vi "TopLevelController.vi"(8 "error in (no error)":errorcluster) -> (0 "error out":errorcluster)   [LabVIEW 2013, in "ToplevelControllerLibrary.lvlib"]
doc: "This Controller controls all interface (User,Display and Sensor )connected to it. New Interfaces can be added."
uses:
  ToplevelControllerLibrary.lvlib
  Modules/DisplayConsole/PrivateContols/DisplayConsole_QueueDriver.ctl
  Modules/UserConsole/PrivateControls/UserConsole_QueueDriver.ctl
  Modules/SensorConsole/PrivateControls/SensorConsole_QueueDriver.ctl
  Modules/Config Database/Private Controls/Queue Driver Control_Config DB.ctl
  Private Controls/Terminate.ctl
  Modules/SensorConsole/SensorConsoleLib.lvlib
  Modules/UserConsole/UserConsole.lvlib
  Modules/DisplayConsole/DisplayConsoleLib.lvlib
  Modules/Config Database/ConfigDBLib.lvlib
panel:
  # "This Controller controls all interface (User,Display and Sensor )connected to it. New Interfaces can be added."
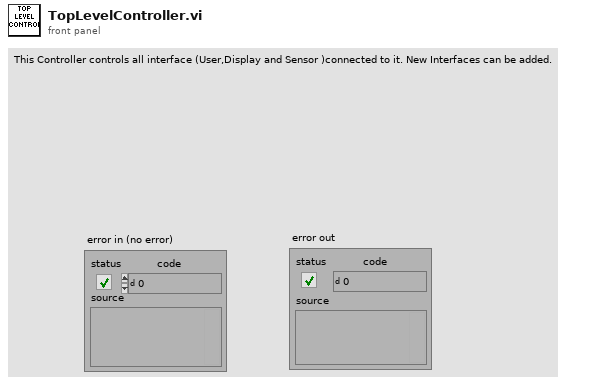
[diagram p1: front panel]
types:
  T1 = enum16{"Init", "Enqueue", "Dequeue", "ReleaseQueue", "Exit"}
  T2 = enum16{"Create Event", "Generate Event", "Destroy Event"}
  T3 = typedef "SensorConsoleLib.lvlib/SensorConsole_QueueDriver.ctl" = enum16{"Default case", "Init", "Enqueue", "Dequeue", "ReleaseQueue", "Exit"}
  T4 = typedef "UserConsole.lvlib/UserConsole_QueueDriver.ctl" = enum16{"Default Case", "Init", "Enqueue", "Dequeue", "ReleaseQueue", "Exit"}
  T5 = typedef "DisplayConsoleLib.lvlib/DisplayConsole_QueueDriver.ctl" = enum16{"Default Case", "Init", "Enqueue", "Dequeue", "ReleaseQueue", "Exit"}
  T6 = typedef "ConfigDBLib.lvlib/Queue Driver Control_Config DB.ctl" = enum16{"Init", "Enqueue", "Dequeue", "ReleaseQueue", "Exit"}
  T7 = typedef "ToplevelControllerLibrary.lvlib/Terminate.ctl" = enum16{"Update UserConsole", "Update DisplayConsole", "ReInit"}
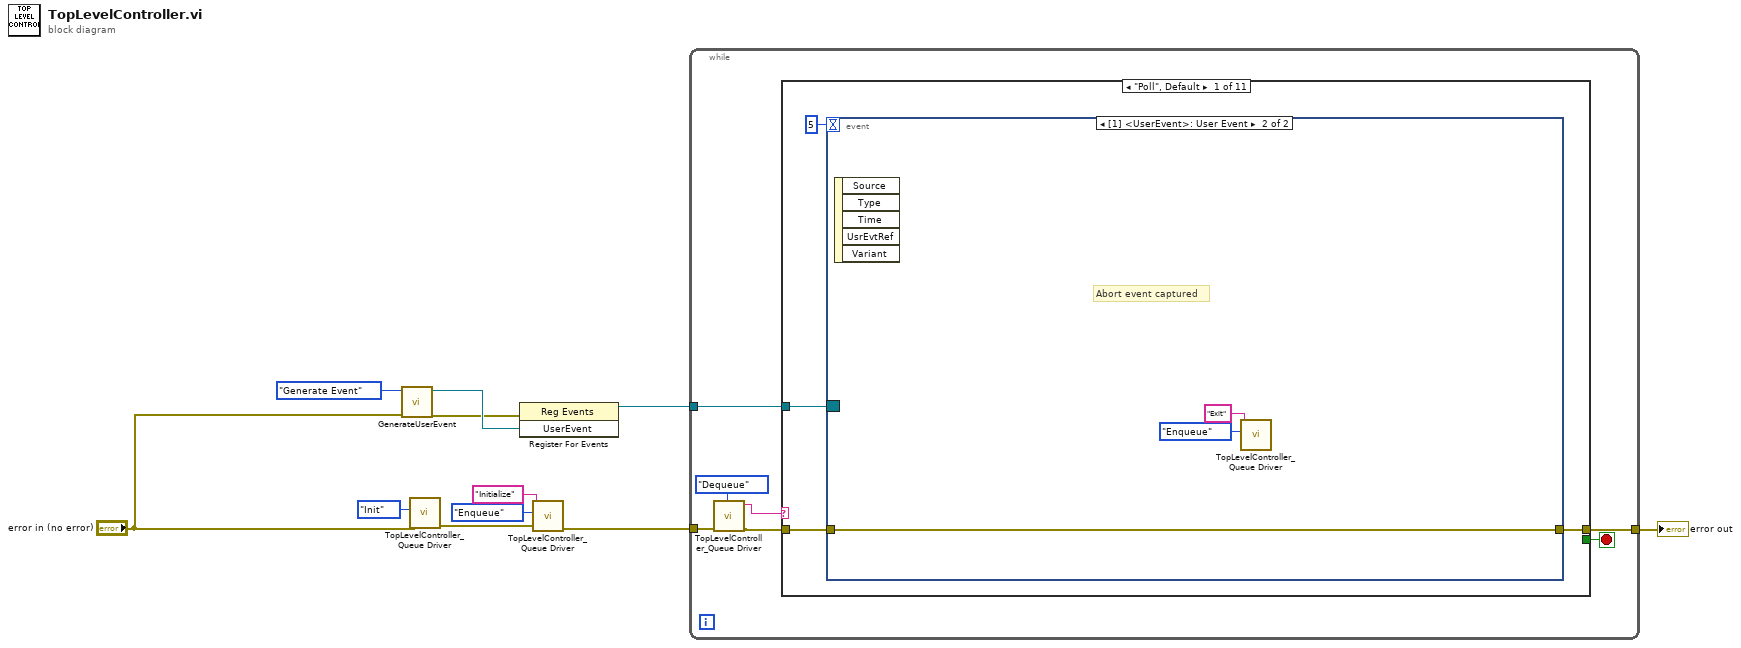
[diagram p0: block diagram]
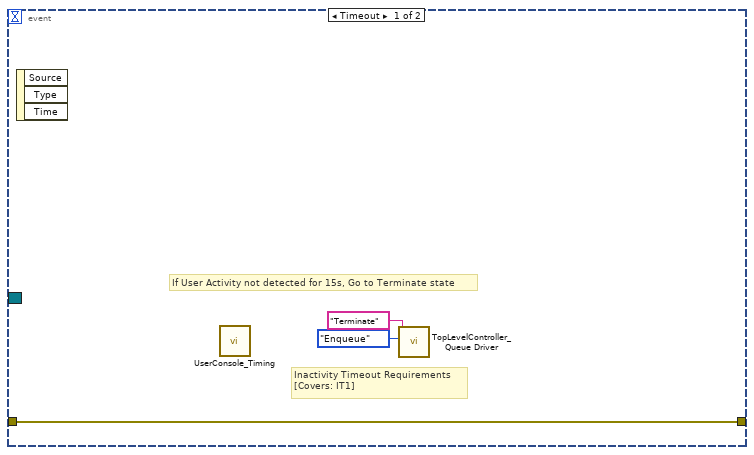
[diagram p2: hidden frame]
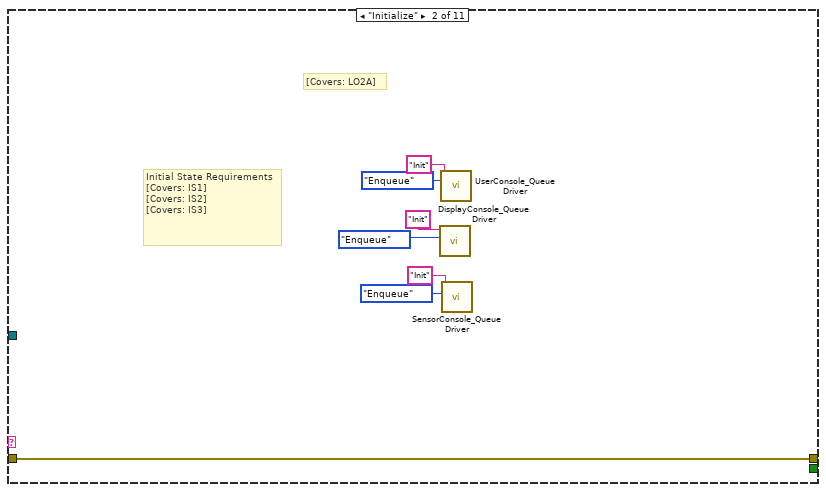
[diagram p3: hidden frame]
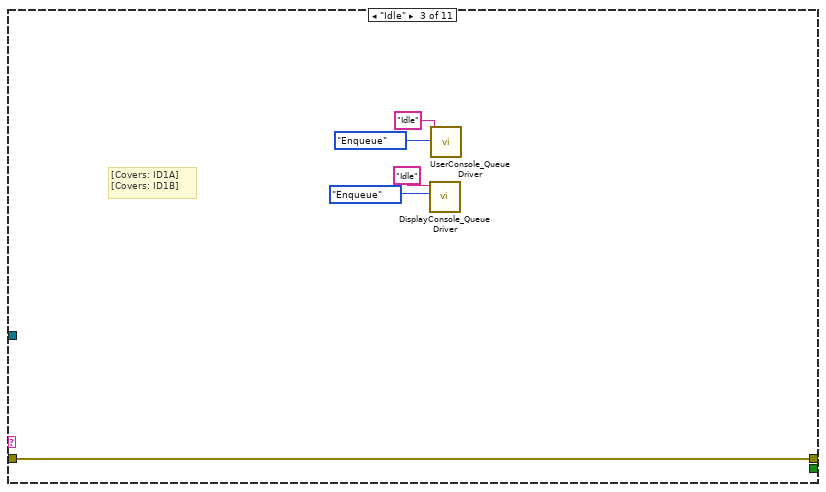
[diagram p4: hidden frame]
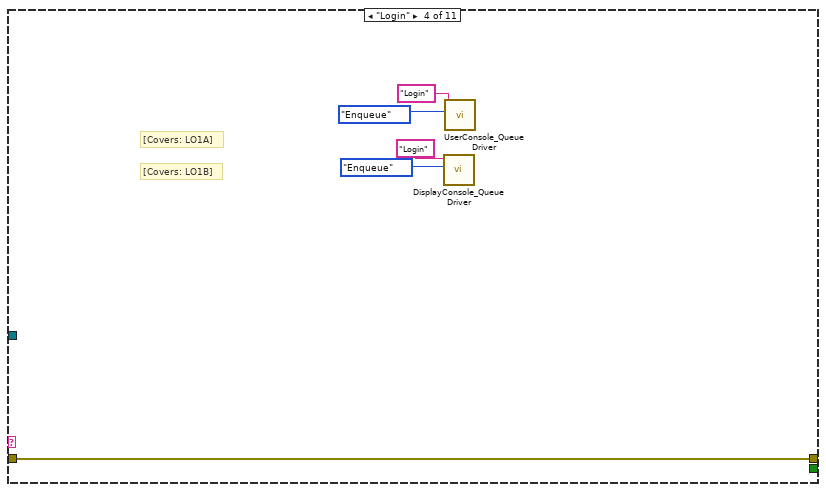
[diagram p5: hidden frame]
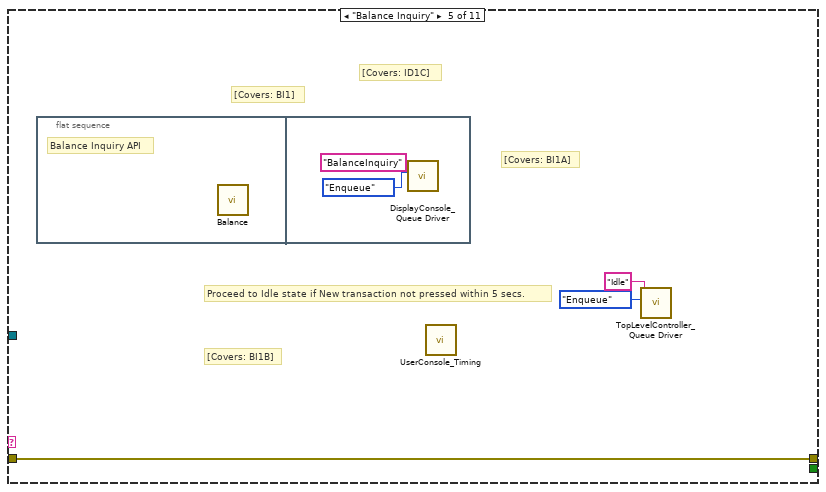
[diagram p6: hidden frame]
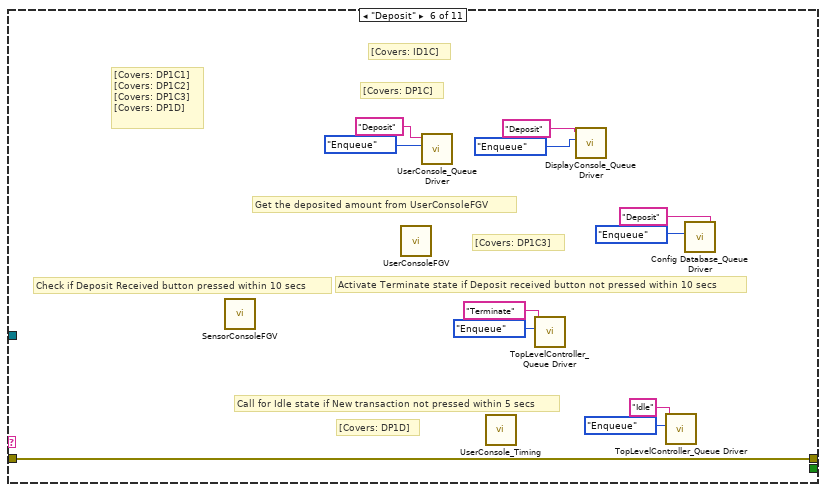
[diagram p7: hidden frame]
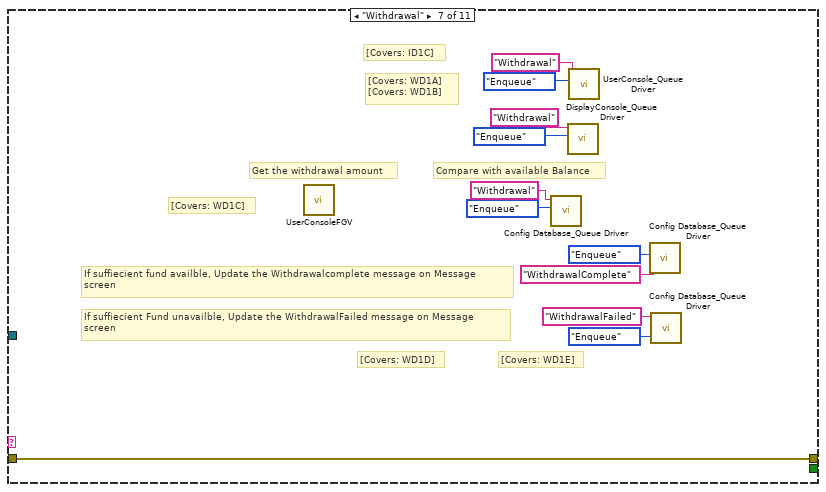
[diagram p8: hidden frame]
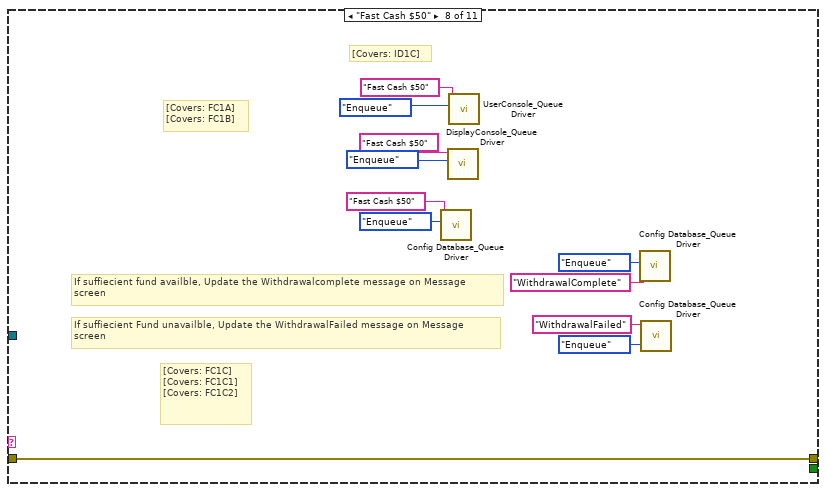
[diagram p9: hidden frame]
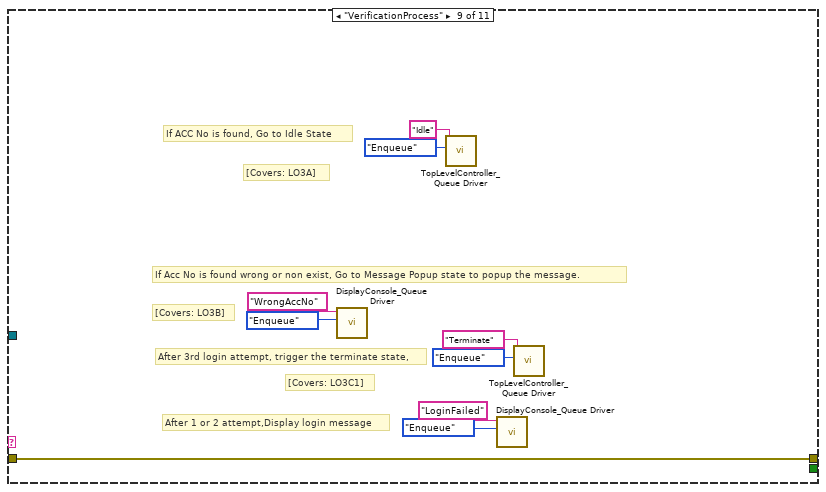
[diagram p10: hidden frame]
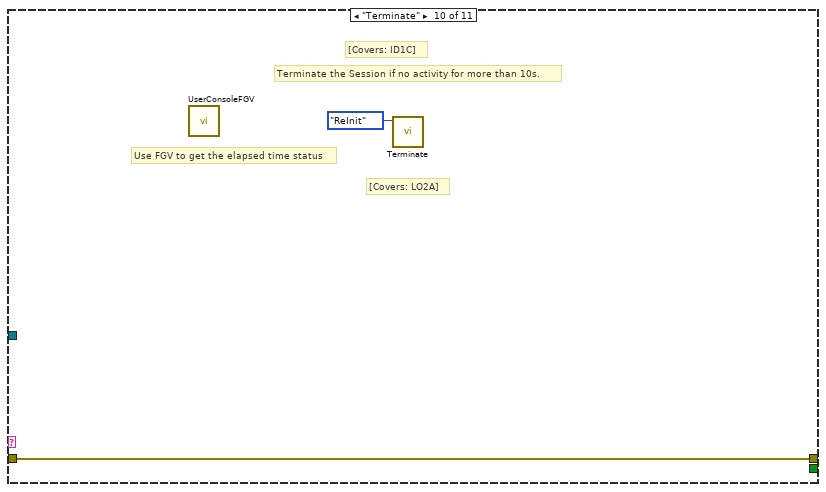
[diagram p11: hidden frame]
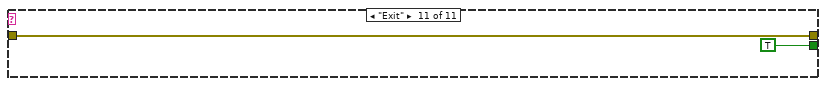
[diagram p12: hidden frame]
diagram:
  n1 = call "GenerateUserEvent.vi"("error in (no error)"="error in (no error)", "Event Actions"=T2."Generate Event") -> ("error out"=w8:errorcluster, "UserEvent"=w10:refnum<user-event>)  [unwired: 8 in]
  n2 = call "TopLevelController_Queue Driver.vi"("error in (no error)"="error in (no error)", "Enum"=T1."Init") -> ("error out"=w6:errorcluster)  [unwired: 8 in, 1 out]
  n3 = register-events(error in=w8, w10) -> (reference out=w9:refnum<event-registration>)  [unwired: 1 in, 1 out]
  n4 = call "TopLevelController_Queue Driver.vi"("error in (no error)"=w6, "Enum"=T1."Enqueue", "EnQ"="Initialize") -> ("error out"=w7:errorcluster)  [unwired: 7 in, 1 out]
  n5 = while {
    tunnel: w9 -> [w18]
    tunnel: w7 -> [w16]
    tunnel: [w13] -> w2
    stop <- w12 stop-if-true
    n6 = call "TopLevelController_Queue Driver.vi"("error in (no error)"=w16, "Enum"=T1."Dequeue") -> ("error out"=w17:errorcluster, "DeQ"=w14:string)  [unwired: 8 in]
    n7 = case shown="\"Poll\", Default" w14 {
      tunnel: w17 -> [w19 w35 w40 w45 w48 w56 w72 w83 w92 w94 w96]
      tunnel: [w20 w35 w40 w45 w48 w56 w72 w83 w92 w94 w96] -> w13
      tunnel: w18 -> [w22 _ _ _ _ _ _ _ _ _ _]
      tunnel: [_ _ _ _ _ _ _ _ _ _ TRUE] -> w12
      frame "Poll", Default {
        n8 = event shown="[1] <UserEvent>: User Event" {
          selector: w22 -> [_ _]
          dyn-events: _ -> [_ _]
          timeout: 5 -> [_ _]
          tunnel: [w23 w28] -> w20
          tunnel: w19 -> [w23 w28]
          event Timeout {
            # "Inactivity Timeout Requirements\n[Covers: IT1]"
            # "If User Activity not detected for 15s, Go to Terminate state"
            n9 = event-data() -> ()  [unwired: 1 in, 3 out]
            n10 = call "UserConsole_Timing.vi"() -> ()  [unwired: 11 in, 1 out]
            n11 = call "TopLevelController_Queue Driver.vi"("Enum"=T1."Enqueue", "EnQ"="Terminate") -> ()  [unwired: 8 in, 2 out]
          }
          event User Event {
            # "Abort event captured"
            n12 = event-data() -> ()  [unwired: 1 in, 5 out]
            n13 = call "TopLevelController_Queue Driver.vi"("Enum"=T1."Enqueue", "EnQ"="Exit") -> ()  [unwired: 8 in, 2 out]
          }
        }
      }
      frame "Initialize" {
        # "Initial State Requirements\n[Covers: IS1]\n[Covers: IS2] \n[Covers: IS3]"
        # "[Covers: LO2A]"
        n14 = call "DisplayConsole_Queue Driver.vi"("State"=DisplayConsole_QueueDriver."Enqueue", "EnQ"="Init") -> ()  [unwired: 8 in, 2 out]
        n15 = call "UserConsole_Queue Driver.vi"("State"=UserConsole_QueueDriver."Enqueue", "EnQ"="Init") -> ()  [unwired: 8 in, 2 out]
        n16 = call "SensorConsole_Queue Driver.vi"("Enum"=SensorConsole_QueueDriver."Enqueue", "EnQ"="Init") -> ()  [unwired: 8 in, 2 out]
      }
      frame "Idle" {
        # "[Covers: ID1A]   \n[Covers: ID1B]"
        n17 = call "DisplayConsole_Queue Driver.vi"("State"=DisplayConsole_QueueDriver."Enqueue", "EnQ"="Idle") -> ()  [unwired: 8 in, 2 out]
        n18 = call "UserConsole_Queue Driver.vi"("State"=UserConsole_QueueDriver."Enqueue", "EnQ"="Idle") -> ()  [unwired: 8 in, 2 out]
      }
      frame "Login" {
        # "[Covers: LO1A]"
        # "[Covers: LO1B]"
        n19 = call "DisplayConsole_Queue Driver.vi"("State"=DisplayConsole_QueueDriver."Enqueue", "EnQ"="Login") -> ()  [unwired: 8 in, 2 out]
        n20 = call "UserConsole_Queue Driver.vi"("State"=UserConsole_QueueDriver."Enqueue", "EnQ"="Login") -> ()  [unwired: 8 in, 2 out]
      }
      frame "Balance Inquiry" {
        # "[Covers: BI1A]"
        # "[Covers: BI1B]"
        # "Proceed to Idle state if New transaction not pressed within 5 secs."
        # "[Covers: BI1]"
        # "[Covers: ID1C]"
        n21 = flat-sequence {
          frame #0 {
            # "Balance Inquiry API"
            n22 = call "Balance.vi"() -> ()  [unwired: 12 in]
          }
          frame #1 {
            n23 = call "DisplayConsole_Queue Driver.vi"("State"=DisplayConsole_QueueDriver."Enqueue", "EnQ"="BalanceInquiry") -> ()  [unwired: 8 in, 2 out]
          }
        }
        n24 = call "UserConsole_Timing.vi"() -> ()  [unwired: 11 in, 1 out]
        n25 = call "TopLevelController_Queue Driver.vi"("Enum"=T1."Enqueue", "EnQ"="Idle") -> ()  [unwired: 8 in, 2 out]
      }
      frame "Deposit" {
        # "[Covers: DP1D]"
        # "Call for Idle state if New transaction not pressed within 5 secs"
        # "[Covers: DP1C3]"
        # "[Covers: DP1C1] \n[Covers: DP1C2] \n[Covers: DP1C3] \n[Covers: DP1D]"
        # "Activate Terminate state if Deposit received button not pressed within 10 secs"
        # "Check if Deposit Received button pressed within 10 secs"
        # "Get the deposited amount from UserConsoleFGV"
        # "[Covers: DP1C]"
        # "[Covers: ID1C]"
        n26 = call "SensorConsoleFGV.vi"() -> ()  [unwired: 10 in, 2 out]
        n27 = call "UserConsoleFGV.vi"() -> ()  [unwired: 10 in, 2 out]
        n28 = call "UserConsole_Queue Driver.vi"("State"=UserConsole_QueueDriver."Enqueue", "EnQ"="Deposit") -> ()  [unwired: 8 in, 2 out]
        n29 = call "UserConsole_Timing.vi"() -> ()  [unwired: 11 in, 1 out]
        n30 = call "TopLevelController_Queue Driver.vi"("Enum"=T1."Enqueue", "EnQ"="Terminate") -> ()  [unwired: 8 in, 2 out]
        n31 = call "DisplayConsole_Queue Driver.vi"("State"=DisplayConsole_QueueDriver."Enqueue", "EnQ"="Deposit") -> ()  [unwired: 8 in, 2 out]
        n32 = call "TopLevelController_Queue Driver.vi"("Enum"=T1."Enqueue", "EnQ"="Idle") -> ()  [unwired: 8 in, 2 out]
        n33 = call "Config Database_Queue Driver.vi"("Enum"=T1."Enqueue", "EnQ"="Deposit") -> ()  [unwired: 8 in, 2 out]
      }
      frame "Withdrawal" {
        # "[Covers: WD1E]"
        # "If suffiecient Fund unavailble, Update the WithdrawalFailed message on Message\nscreen"
        # "[Covers: WD1D]"
        # "If suffiecient fund availble, Update the Withdrawalcomplete message on Message\nscreen"
        # "[Covers: WD1C]"
        # "Compare with available Balance"
        # "Get the withdrawal amount"
        # "[Covers: WD1A]  \n[Covers: WD1B]"
        # "[Covers: ID1C]"
        n34 = call "UserConsoleFGV.vi"() -> ()  [unwired: 10 in, 2 out]
        n35 = call "Config Database_Queue Driver.vi"("Enum"=T1."Enqueue", "EnQ"="Withdrawal") -> ()  [unwired: 8 in, 2 out]
        n36 = call "DisplayConsole_Queue Driver.vi"("State"=DisplayConsole_QueueDriver."Enqueue", "EnQ"="Withdrawal") -> ()  [unwired: 8 in, 2 out]
        n37 = call "UserConsole_Queue Driver.vi"("State"=UserConsole_QueueDriver."Enqueue", "EnQ"="Withdrawal") -> ()  [unwired: 8 in, 2 out]
        n38 = call "Config Database_Queue Driver.vi"("Enum"=Queue_Driver_Control_Config_DB."Enqueue", "EnQ"="WithdrawalComplete") -> ()  [unwired: 8 in, 2 out]
        n39 = call "Config Database_Queue Driver.vi"("Enum"=Queue_Driver_Control_Config_DB."Enqueue", "EnQ"="WithdrawalFailed") -> ()  [unwired: 8 in, 2 out]
      }
      frame "Fast Cash $50" {
        # "[Covers: FC1C] \n[Covers: FC1C1] \n[Covers: FC1C2]"
        # "If suffiecient Fund unavailble, Update the WithdrawalFailed message on Message\nscreen"
        # "If suffiecient fund availble, Update the Withdrawalcomplete message on Message\nscreen"
        # "[Covers: FC1A] \n[Covers: FC1B]"
        # "[Covers: ID1C]"
        n40 = call "Config Database_Queue Driver.vi"("Enum"=Queue_Driver_Control_Config_DB."Enqueue", "EnQ"="Fast Cash $50") -> ()  [unwired: 8 in, 2 out]
        n41 = call "DisplayConsole_Queue Driver.vi"("State"=DisplayConsole_QueueDriver."Enqueue", "EnQ"="Fast Cash $50") -> ()  [unwired: 8 in, 2 out]
        n42 = call "UserConsole_Queue Driver.vi"("State"=UserConsole_QueueDriver."Enqueue", "EnQ"="Fast Cash $50") -> ()  [unwired: 8 in, 2 out]
        n43 = call "Config Database_Queue Driver.vi"("Enum"=Queue_Driver_Control_Config_DB."Enqueue", "EnQ"="WithdrawalComplete") -> ()  [unwired: 8 in, 2 out]
        n44 = call "Config Database_Queue Driver.vi"("Enum"=Queue_Driver_Control_Config_DB."Enqueue", "EnQ"="WithdrawalFailed") -> ()  [unwired: 8 in, 2 out]
      }
      frame "VerificationProcess" {
        # "After 1 or 2 attempt,Display login message"
        # "[Covers: LO3C1]"
        # "After 3rd login attempt, trigger the terminate state,"
        # "[Covers: LO3B]"
        # "If Acc No is found wrong or non exist, Go to Message Popup state to popup the message."
        # "[Covers: LO3A]"
        # "If ACC No is found, Go to Idle State"
        n45 = call "DisplayConsole_Queue Driver.vi"("State"=DisplayConsole_QueueDriver."Enqueue", "EnQ"="WrongAccNo") -> ()  [unwired: 8 in, 2 out]
        n46 = call "TopLevelController_Queue Driver.vi"("Enum"=T1."Enqueue", "EnQ"="Idle") -> ()  [unwired: 8 in, 2 out]
        n47 = call "DisplayConsole_Queue Driver.vi"("State"=DisplayConsole_QueueDriver."Enqueue", "EnQ"="LoginFailed") -> ()  [unwired: 8 in, 2 out]
        n48 = call "TopLevelController_Queue Driver.vi"("Enum"=T1."Enqueue", "EnQ"="Terminate") -> ()  [unwired: 8 in, 2 out]
      }
      frame "Terminate" {
        # "Use FGV to get the elapsed time status"
        # "[Covers: ID1C]"
        # "[Covers: LO2A]"
        # "Terminate the Session if no activity for more than 10s."
        n49 = call "UserConsoleFGV.vi"() -> ()  [unwired: 10 in, 2 out]
        n50 = call "Terminate.vi"("Terminate"=Terminate."ReInit") -> ()  [unwired: 11 in]
      }
      frame "Exit" {
      }
    }
  }
  "error out" <- w2
